vi "Autonomous Independent.vi"() -> ()   [LabVIEW 2016]
doc: "This VI is called when autonomous begins, and will automatically be terminated when autonomous ends. You can carry out timed or sensor driven robot movement independently without needing to return to the caller."
uses:
  <vilib>/Rock Robotics/WPI/Solenoid/WPI_SolenoidValue.ctl
  <vilib>/Rock Robotics/WPI/Utilities/WPI_GetSetVariantRefNum.vi
  <vilib>/Rock Robotics/Network Tables/NT Write Numeric Array.vi
  <vilib>/Rock Robotics/Network Tables/NT Read String.vi
  <vilib>/Rock Robotics/WPI/Solenoid/WPI_SolenoidSetEnum.vi
  <vilib>/Rock Robotics/WPI/RobotDrive/WPI_RobotDriveMecanumDrive_Cartesian.vi
panel:
  out "Current Movement, for debugging":T1 {"Z Joystick Value" scale=-1.0..1.0; "Y Joystick Value" scale=1.0..-1.0; "X Joystick Value" scale=-1.0..1.0}
  in  "Array of robot movements":T2(array[cluster])=[{"X Joystick Value"=-0.010101010101010017, "Y Joystick Value"=0.0, "Z Joystick Value"=0.4574773480918073, "Delay (sec)"=0.0, "Movement Name"=""}, {"X Joystick Value"=0.050505050505050594, "Y Joystick Value"=0.0, "Z Joystick Value"=-0.25616029503917137, "Delay (sec)"=0.0, "Movement Name"=""}] {"Z Joystick Value" scale=-1.0..1.0; "Y Joystick Value" scale=1.0..-1.0; "X Joystick Value" scale=-1.0..1.0}
  # "Be sure to right-click and choose Data Operations>>Make Current Value default if you want to save the array values with the VI"
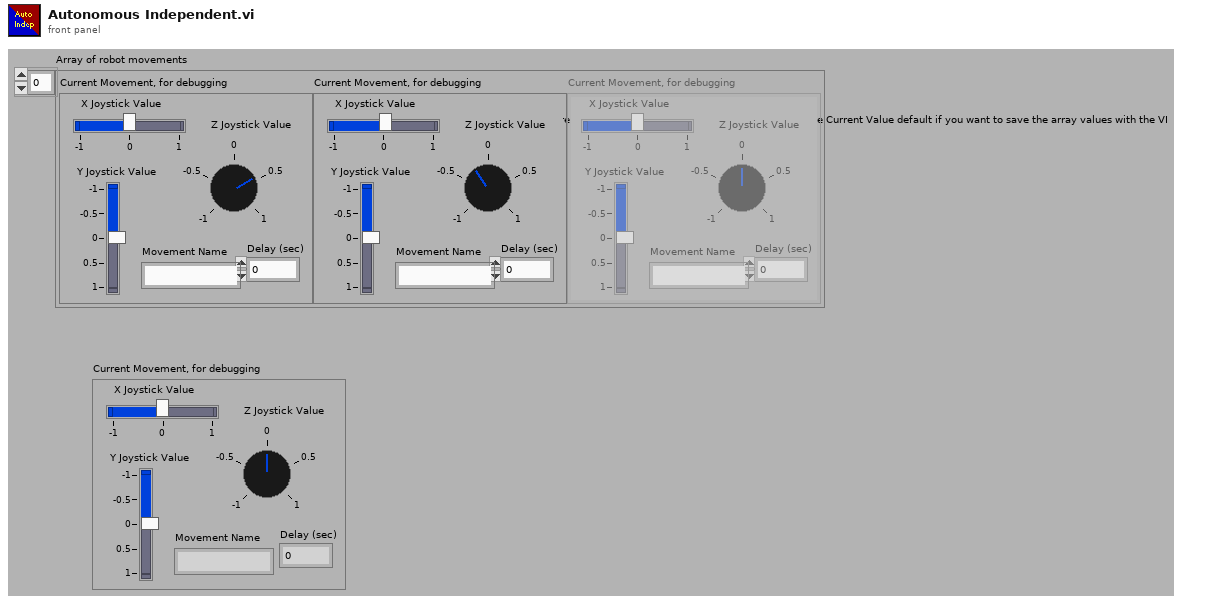
[diagram p1: front panel]
types:
  T1 = cluster{"X Joystick Value":dbl, "Y Joystick Value":dbl, "Z Joystick Value":dbl, "Delay (sec)":dbl, "Movement Name":string}
  T2 = cluster{"X Joystick Value":dbl, "Y Joystick Value":dbl, "Z Joystick Value":dbl, "Delay (sec)":dbl, "Movement Name":string}[]
  T3 = typedef "WPI_JoystickDevRef.ctl" = cluster{"Device":T4}
  T4 = typedef "WPI_JoystickDeviceEnum.ctl" = enum16{"USB 0", "USB 1", "USB 2", "USB 3", "USB 4", "USB 5"}
  T5 = typedef "WPI_SolenoidValue.ctl" = enum16{"Off", "On", "Forward", "Reverse"}
  T6 = typedef "WPI_SolenoidDevRef.ctl" = cluster{"DevStatus":errorcluster, "Pneumatics Control Module":u8, "Forward Solenoid Channel":T7, "Reverse Solenoid Channel":T7}
  T7 = typedef "WPI_SolenoidChannel.ctl" = enum8{"Solenoid 0", "Solenoid 1", "Solenoid 2", "Solenoid 3", "Solenoid 4", "Solenoid 5", "Solenoid 6", "Solenoid 7", "Invalid"}
  T8 = typedef "WPI_RobotDriveDevRef.ctl" = cluster{"DevStatus":errorcluster, "Motors[]":T9[], "Square Inputs":bool, "Max Output":dbl}
  T9 = typedef "WPI_MotorControlDeviceRef.ctl" = cluster{"DeviceStatus":errorcluster, "Type":T10, "PWM":cluster{"PWM Channel":T11, "DeadBand":T12}, "CAN":cluster{"Device Number":u8, "SetOutput VI Ref":variant, "GetOutput VI Ref":variant, "Enable VI Ref":variant, "Disable VI Ref":variant, "Data":variant}, "Invert":bool}
  T10 = typedef "WPI_MotorControlType.ctl" = enum16{"PWM", "CAN"}
  T11 = typedef "FPGA_DIOPWMChannel.ctl" = enum8{"PWM 0", "PWM 1", "PWM 2", "PWM 3", "PWM 4", "PWM 5", "PWM 6", "PWM 7", "PWM 8", "PWM 9", "PWM MXP 0", "PWM MXP 1", "PWM MXP 2", "PWM MXP 3", "PWM MXP 4", "PWM MXP 5", "PWM MXP 6", "PWM MXP 7", "PWM MXP 8", "PWM MXP 9", "Invalid"}
  T12 = typedef "WPI_PWMDeadband.ctl" = cluster{"Name":string, "maxPositivePwm":i32, "minPositivePwm":i32, "centerPwm":i32, "maxNegativePwm":i32, "minNegativePwm":i32, "angularRange":u16}
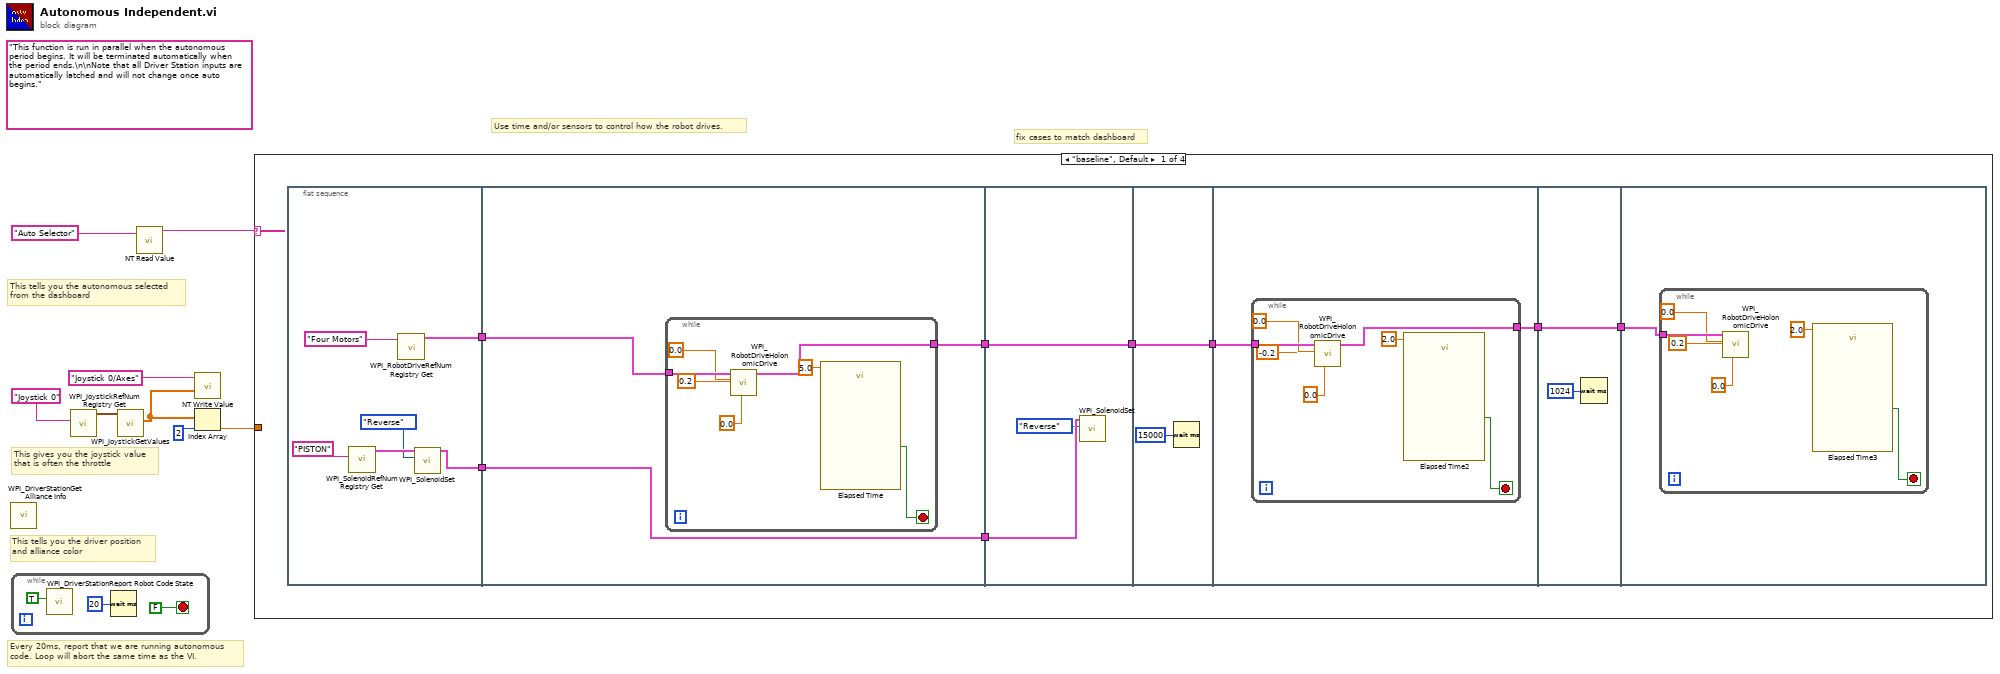
[diagram p0: block diagram]
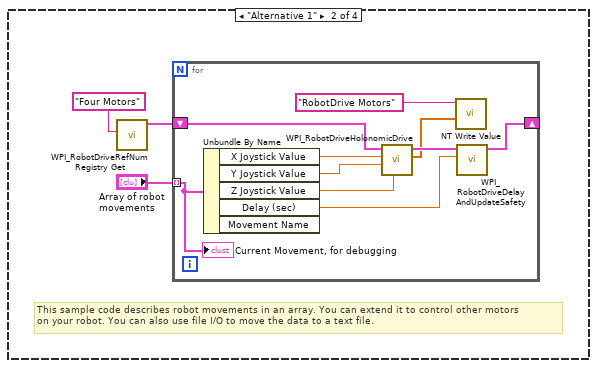
[diagram p2: hidden frame]
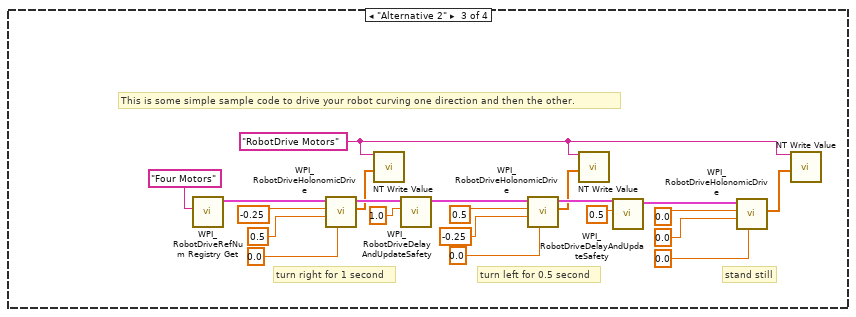
[diagram p3: hidden frame]
diagram:
  (unwired) "This function is run in parallel when the autonomous period begins. It will be terminated automatically when the period ends.\n\nNote that all Driver Station inputs are automatically latched and will not change once auto begins."
  # "fix cases to match dashboard"
  # "This tells you the autonomous selected\nfrom the dashboard"
  # "Every 20ms, report that we are running autonomous\ncode. Loop will abort the same time as the VI."
  # "This gives you the joystick value\nthat is often the throttle"
  # "Use time and/or sensors to control how the robot drives."
  # "This tells you the driver position\nand alliance color"
  n1 = call <vilib>:"WPI_DriverStationGet Alliance Info.vi"() -> ()  [unwired: 12 out]
  n2 = while {
    stop <- FALSE stop-if-true
    n3 = call <vilib>:"WPI_DriverStationReport Robot Code State.vi"("Autonomous"=TRUE) -> ()  [unwired: 10 in, 1 out]
    n4 = Wait (ms)(milliseconds to wait=u32 20) -> ()  [unwired: 1 out]
  }
  n5 = call <vilib>:"WPI_JoystickRefNum Registry Get.vi"("refnum name"="Joystick 0") -> ("JoystickDevRef"=w7:T3)  [unwired: 1 in, 9 out]
  n6 = call <vilib>:"WPI_JoystickGetValues.vi"("JoystickDevRef"=w7) -> ("Axes"=w3:dbl[])  [unwired: 6 in, 4 out]
  n7 = call-poly <vilib>:"NT Read Value.vi"("Name"="Auto Selector") -> ("String"=w2:string)  [unwired: 9 in, 1 out]
  n8 = call-poly <vilib>:"NT Write Value.vi"("Numeric Array"=w3, "Name"="Joystick 0/Axes") -> ()  [unwired: 9 in, 1 out]
  n9 = Index Array(array=w3, index=u32 2 ("milliseconds to wait")) -> (element=w1:dbl)
  n10 = case shown="\"baseline\", Default" w2 {
    tunnel: w1 -> [_ _ _ _]
    frame "baseline", Default {
      n11 = flat-sequence {
        tunnel: [w22] -> w18
        tunnel: [w20] -> w17
        tunnel: [w28] -> w19
        tunnel: w18 -> [w28]
        tunnel: w17 -> [w27]
        tunnel: [w26] -> w16
        tunnel: w19 -> [w38]
        tunnel: w16 -> [w36]
        tunnel: [w36] -> w15
        tunnel: w15 -> [w39]
        tunnel: [w39] -> w14
        tunnel: w14 -> [w42]
        tunnel: [w41] -> w13
        tunnel: w13 -> [w50]
        tunnel: [w50] -> w12
        tunnel: w12 -> [w52]
        frame #0 {
          n12 = call <vilib>:"WPI_SolenoidRefNum Registry Get.vi"("refnum name"="PISTON") -> ("SolenoidDevRef"=w25:T6)  [unwired: 9 in, 1 out]
          n13 = call <vilib>:"WPI_RobotDriveRefNum Registry Get.vi"("refnum name"="Four Motors") -> ("RobotDriveDevRef"=w20:T8)  [unwired: 9 in, 1 out]
          n14 = call-poly <vilib>:"WPI_SolenoidSet.vi"("Value"=WPI_SolenoidValue."Reverse", "SolenoidDevRef"=w25) -> ("SolenoidDevRef"=w22:T6)  [unwired: 8 in, 1 out]
        }
        frame #1 {
          n15 = while {
            tunnel: w27 -> [w35]
            tunnel: [w29] -> w26
            stop <- w30 stop-if-true
            n16 = call-poly <vilib>:"WPI_RobotDriveHolonomicDrive.vi"("Rotation"=0.0, "Y"=0.2, "X"=0.0, "RobotDriveDevRef"=w35) -> ("RobotDriveDevRef"=w29:T8)  [unwired: 5 in, 2 out]
            n17 = call "Elapsed Time"("Time Target (s)"=5.0) -> ("Time has Elapsed"=w30:bool)  [unwired: 11 in, 7 out]
          }
        }
        frame #2 {
          n18 = call-poly <vilib>:"WPI_SolenoidSet.vi"("Value"=WPI_SolenoidValue."Reverse", "SolenoidDevRef"=w38) -> ()  [unwired: 8 in, 2 out]
        }
        frame #3 {
          n19 = Wait (ms)(milliseconds to wait=u32 15000) -> ()  [unwired: 1 out]
        }
        frame #4 {
          n20 = while {
            tunnel: w42 -> [w49]
            tunnel: [w43] -> w41
            stop <- w44 stop-if-true
            n21 = call-poly <vilib>:"WPI_RobotDriveHolonomicDrive.vi"("Rotation"=0.0, "Y"=-0.2, "X"=0.0, "RobotDriveDevRef"=w49) -> ("RobotDriveDevRef"=w43:T8)  [unwired: 5 in, 2 out]
            n22 = call "Elapsed Time2"("Time Target (s)"=2.0) -> ("Time has Elapsed"=w44:bool)  [unwired: 11 in, 7 out]
          }
        }
        frame #5 {
          n23 = Wait (ms)(milliseconds to wait=u32 1024) -> ()  [unwired: 1 out]
        }
        frame #6 {
          n24 = while {
            tunnel: w52 -> [w58]
            stop <- w53 stop-if-true
            n25 = call-poly <vilib>:"WPI_RobotDriveHolonomicDrive.vi"("Rotation"=0.0, "Y"=0.2, "X"=0.0, "RobotDriveDevRef"=w58) -> ()  [unwired: 5 in, 3 out]
            n26 = call "Elapsed Time3"("Time Target (s)"=2.0) -> ("Time has Elapsed"=w53:bool)  [unwired: 11 in, 7 out]
          }
        }
      }
    }
    frame "Alternative 1" {
      # "This sample code describes robot movements in an array. You can extend it to control other motors\non your robot. You can also use file I/O to move the data to a text file."
      n27 = call <vilib>:"WPI_RobotDriveRefNum Registry Get.vi"("refnum name"="Four Motors") -> ("RobotDriveDevRef"=w60:T8)  [unwired: 1 in, 9 out]
      n28 = for {
        shift-right: [w69] -> _
        shift-left: w60 -> [w70]
        tunnel: "Array of robot movements" -> [w65] mode=indexing
        n29 = Unbundle By Name(w65) -> ("X Joystick Value"=w68:dbl, "Y Joystick Value"=w67:dbl, "Z Joystick Value"=w64:dbl, "Delay (sec)"=w66:dbl)  [unwired: 1 out]
        n30 = call-poly <vilib>:"WPI_RobotDriveHolonomicDrive.vi"("Rotation"=w64, "Y"=w67, "X"=w68, "RobotDriveDevRef"=w70) -> ("Motor Values"=w62:dbl[], "RobotDriveDevRef"=w71:T8)  [unwired: 5 in, 1 out]
        n31 = call-poly <vilib>:"NT Write Value.vi"("Numeric Array"=w62, "Name"="RobotDrive Motors") -> ()  [unwired: 9 in, 1 out]
        n32 = call <vilib>:"WPI_RobotDriveDelayAndUpdateSafety.vi"("Delay (s)"=w66, "RobotDriveDevRef"=w71) -> ("RobotDriveDevRef 2"=w69:T8)  [unwired: 8 in, 1 out]
        "Current Movement, for debugging" <- w65
      }
    }
    frame "Alternative 2" {
      w72 = "RobotDrive Motors" ("Name")
      # "This is some simple sample code to drive your robot curving one direction and then the other."
      # "stand still"
      # "turn left for 0.5 second"
      # "turn right for 1 second"
      n33 = call <vilib>:"WPI_RobotDriveRefNum Registry Get.vi"("refnum name"="Four Motors") -> ("RobotDriveDevRef"=w89:T8)  [unwired: 1 in, 9 out]
      n34 = call-poly <vilib>:"WPI_RobotDriveHolonomicDrive.vi"("Rotation"=0.0, "Y"=0.5 ("X axis value"), "X"=-0.25 ("X axis value"), "RobotDriveDevRef"=w89) -> ("Motor Values"=w73:dbl[], "RobotDriveDevRef"=w82:T8)  [unwired: 5 in, 1 out]
      n35 = call-poly <vilib>:"NT Write Value.vi"("Numeric Array"=w73, "Name"=w72) -> ()  [unwired: 9 in, 1 out]
      n36 = call <vilib>:"WPI_RobotDriveDelayAndUpdateSafety.vi"("Delay (s)"=1.0, "RobotDriveDevRef"=w82) -> ("RobotDriveDevRef 2"=w83:T8)  [unwired: 8 in, 1 out]
      n37 = call-poly <vilib>:"WPI_RobotDriveHolonomicDrive.vi"("Rotation"=0.0, "Y"=-0.25 ("X axis value"), "X"=0.5 ("X axis value"), "RobotDriveDevRef"=w83) -> ("Motor Values"=w74:dbl[], "RobotDriveDevRef"=w84:T8)  [unwired: 5 in, 1 out]
      n38 = call-poly <vilib>:"NT Write Value.vi"("Numeric Array"=w74, "Name"=w72) -> ()  [unwired: 9 in, 1 out]
      n39 = call <vilib>:"WPI_RobotDriveDelayAndUpdateSafety.vi"("Delay (s)"=0.5, "RobotDriveDevRef"=w84) -> ("RobotDriveDevRef 2"=w85:T8)  [unwired: 8 in, 1 out]
      n40 = call-poly <vilib>:"WPI_RobotDriveHolonomicDrive.vi"("Rotation"=0.0 ("X axis value"), "Y"=0.0 ("X axis value"), "X"=0.0 ("X axis value"), "RobotDriveDevRef"=w85) -> ("Motor Values"=w75:dbl[])  [unwired: 5 in, 2 out]
      n41 = call-poly <vilib>:"NT Write Value.vi"("Numeric Array"=w75, "Name"=w72) -> ()  [unwired: 9 in, 1 out]
    }
    frame "Your Turn" {
    }
  }
